vi "Restore Menu.vi"(8 "error in (no error)":errorcluster, 9 "Menu ref":refnum<vi>, 10 "File path":path, 11 "Monitor-Pulse in":refnum<class "Application Controller.lvclass">) -> (0 "error out":errorcluster, 1 "Section out":string, 2 "File path out":path, 3 "Monitor-Pulse out":refnum<class "Application Controller.lvclass">)   [LabVIEW 2019, in "Application Controller.lvclass"]
uses:
  Application Controller.lvclass
  C:/GitHub/LabActor/Template Module/Template Module.lvclass
  NHMFL_Core/Libraries/Queued Listbox/Queued Listbox.xctl
  Template Module/Template Module.lvclass/Template Module.ctl
  Template Module/Read Name.vi
  <vilib>/Utility/error.llb/Error Cluster From Error Code.vi
  <vilib>/ErrorRing/Error Ring.xnode
  <vilib>/Utility/config.llb/NI_LVConfig.lvlib
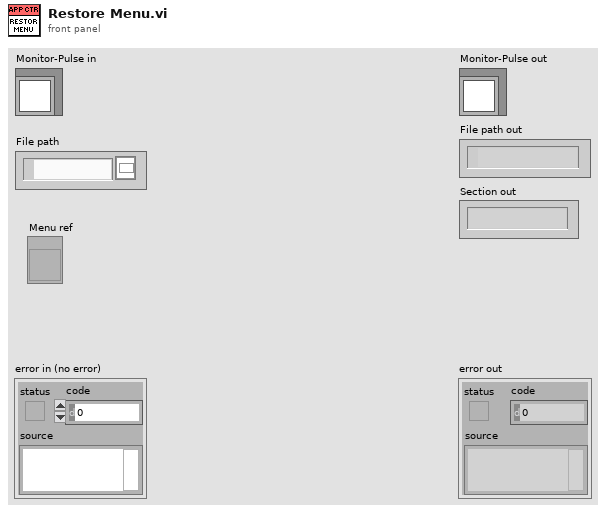
[diagram p1: front panel]
types:
  T1 = typedef "NI_LVConfig.lvlib/Config Data RefNum.ctl" = refnum<k1>
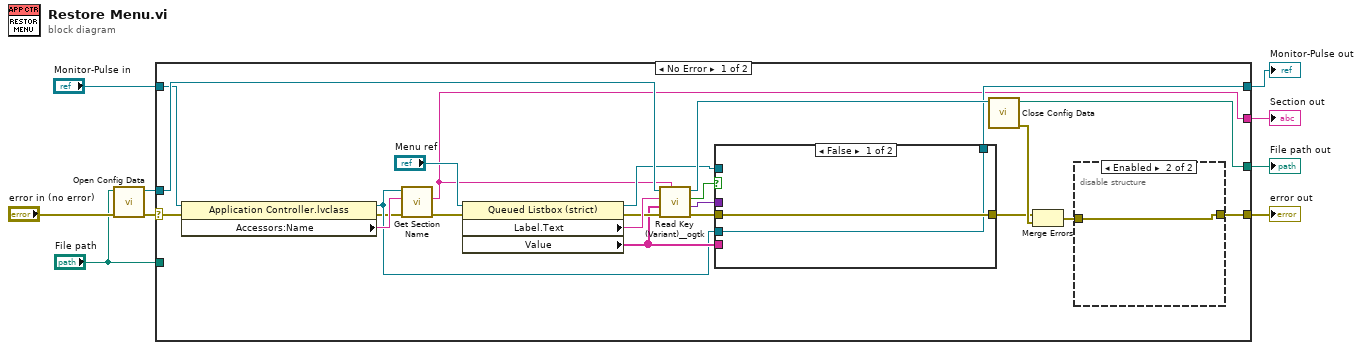
[diagram p0: block diagram]
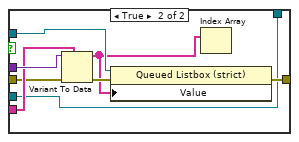
[diagram p2: hidden frame]
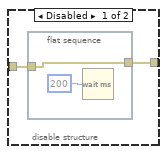
[diagram p3: hidden frame]
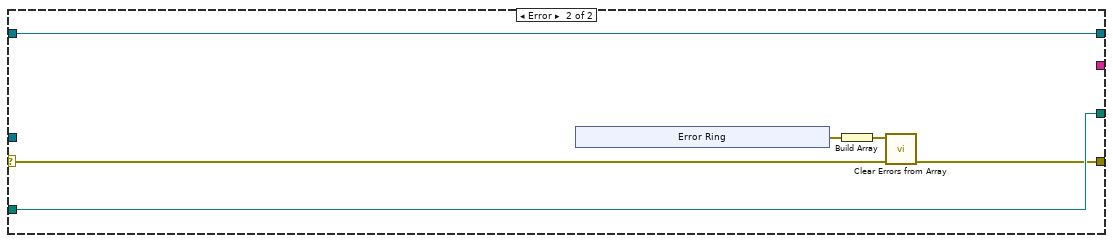
[diagram p4: hidden frame]
diagram:
  n1 = call <vilib>:"Open Config Data.vi"("error in (no error)"="error in (no error)", "configuration file path"="File path") -> ("error out"=w2:errorcluster, "refnum"=w9:T1)  [unwired: 7 in, 1 out]
  n2 = case shown="No Error" w2 {
    selector: w2 -> [w23 w49]
    tunnel: w9 -> [w32 _]
    tunnel: [w11 _] -> w8
    tunnel: [w13 w53] -> w7
    tunnel: "Monitor-Pulse in" -> [w27 w53]
    tunnel: [w15 w48] -> w5
    tunnel: [w25 w52] -> w4
    tunnel: "File path" -> [_ w52]
    frame No Error {
      n3 = property class="Application Controller.lvclass"(reference=w27, error in=w23) -> (reference out=w12:refnum<class "Application Controller.lvclass">, error out=w10:errorcluster, "Accessors:Name"=w14:string)
      n4 = call "Get Section Name.vi"("Error In"=w10, "Object name"=w14, "object"=w12) -> ("Error Out"=w24:errorcluster, "Section out"=w11:string)  [unwired: 7 in]
      n5 = property class="Queued Listbox (strict)"(reference="Menu ref", error in=w24) -> (reference out=w20:refnum<vi>, error out=w21:errorcluster, "Label.Text"=w28:string, "Value"=w18:string[])
      n6 = call <userlib>:"Read Key (Variant)__ogtk.vi"("section"=w11, "error in (no error)"=w21, "type"=w18, "key (optional)"=w28, "refnum"=w32) -> ("error out"=w17:errorcluster, "key-value"=w19:variant, "found?"=w16:bool, "refnum out"=w29:T1)  [unwired: 3 in]
      n7 = case shown="False" w16 {
        tunnel: w20 -> [_ w42]
        tunnel: w19 -> [_ w41]
        tunnel: w18 -> [_ w40]
        tunnel: w17 -> [w34 w39]
        tunnel: [w34 w37] -> w30
        tunnel: w12 -> [w33 w36]
        tunnel: [w33 w36] -> w13
        frame False {
        }
        frame True {
          n8 = Variant To Data(error in=w39, type=w40, Variant=w41) -> (data=w35:string[], error out=w38:errorcluster)
          n9 = property class="Queued Listbox (strict)"(reference=w42, error in=w38, "Value"=w35) -> (error out=w37:errorcluster)  [unwired: 1 out]
          n10 = Index Array(array=w35) -> ()  [unwired: 1 in, 1 out]
        }
      }
      n11 = call <vilib>:"Close Config Data.vi"("refnum"=w29) -> ("error out"=w31:errorcluster, "file path"=w25:path)  [unwired: 9 in]
      n12 = Merge Errors(w30, w31) -> (w26:errorcluster)
      n13 = disable-structure shown="Enabled" {
        disable-tunnel: w26 -> [w44 w47]
        disable-tunnel: [w43 w47] -> w15
        frame Disabled {
          n14 = flat-sequence {
            tunnel: w44 -> [w46]
            tunnel: [w46] -> w43
            frame #0 {
              n15 = Wait (ms)(milliseconds to wait=u32 200) -> ()  [unwired: 1 out]
            }
          }
        }
        frame Enabled {
        }
      }
    }
    frame Error {
      n16 = xnode "Error Ring"() -> ("error out"=w51:errorcluster)
      n17 = Build Array(w51) -> (w50:errorcluster[])
      n18 = call "Clear Errors from Array.vi"("Error In"=w49, "Errors to clear"=w50) -> ("Error Out"=w48:errorcluster)  [unwired: 8 in, 1 out]
    }
  }
  "error out" <- w5
  "Monitor-Pulse out" <- w7
  "File path out" <- w4
  "Section out" <- w8
